vi "Globals.vi"() -> ()   [LabVIEW 2017, in "LabPack.lvlib"]
uses:
  LabPack.lvlib
panel:
  in  "Shared Library":path=path ""
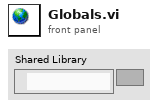
[diagram p1: front panel]
diagram:
